vi "Controller - Fire Message.vi"(8 "error in (no error)":errorcluster, 10 "Message Name":T1, 11 "View Model":T2) -> (0 "error out":errorcluster, 3 "View Model":T2)   [LabVIEW 2017]
doc: "Fire message user event with parameters"
uses:
  View Model/Controls/View Model.ctl
  Error Handler/Controls/Error Model.ctl
  Error Handler/Controls/Error Data.ctl
  Error Handler/Controls/Error Type.ctl
  View Model/Controls/Shared Model.ctl
  Configuration/Controls/Config Model.ctl
  Configuration/Controls/Config CMD.ctl
  Configuration/Controls/Config Data.ctl
  Controls/Controller Model.ctl
  Controls/Controller Overhead.ctl
  Controls/Controller States.ctl
  Controls/Controller Message Data.ctl
  Controls/Controller Message Name.ctl
  Views/User Console View/Controls/User Console - Keypad.ctl
  Views/User Console View/Controls/User Console - Transactions.ctl
  Controls/Controller CMD.ctl
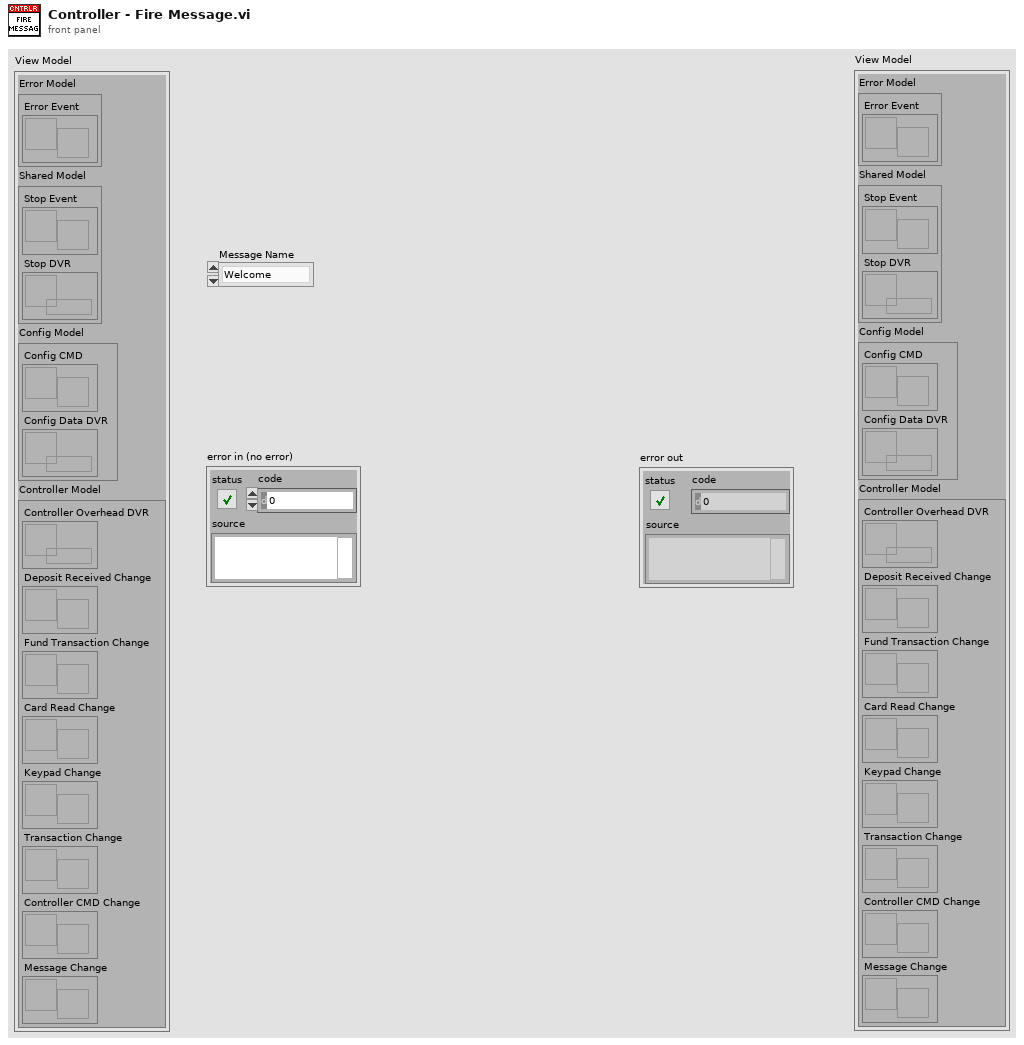
[diagram p1: front panel]
types:
  T1 = typedef "Controller Message Name.ctl" = enum16{"Welcome", "Login", "Idle", "Invalid Login", "Terminate", "Deposit", "Withdrawal", "Fast Cash", "Withdrawal Complete", "Withdrawal Failed", "Balance Inquiry"}
  T2 = typedef "View Model.ctl" = cluster{"Error Model":T3, "Shared Model":T4, "Config Model":T5, "Controller Model":T6}
  T3 = typedef "Error Model.ctl" = cluster{"Error Event":refnum<user-event>}
  T4 = typedef "Shared Model.ctl" = cluster{"Stop Event":refnum<user-event>, "Stop DVR":refnum<data-value>}
  T5 = typedef "Config Model.ctl" = cluster{"Config CMD":refnum<user-event>, "Config Data DVR":refnum<data-value>}
  T6 = typedef "Controller Model.ctl" = cluster{"Controller Overhead DVR":refnum<data-value>, "Deposit Received Change":refnum<user-event>, "Fund Transaction Change":refnum<user-event>, "Card Read Change":refnum<user-event>, "Keypad Change":refnum<user-event>, "Transaction Change":refnum<user-event>, "Controller CMD Change":refnum<user-event>, "Message Change":refnum<user-event>}
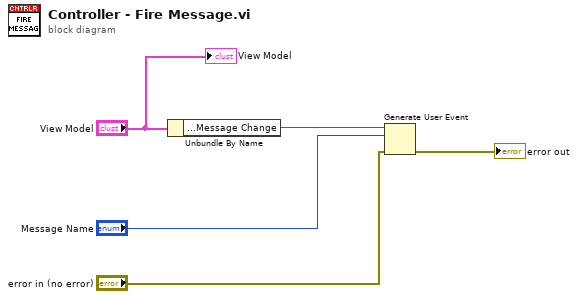
[diagram p0: block diagram]
diagram:
  n1 = Unbundle By Name("View Model") -> ("Controller Model.Message Change"=w5:refnum<user-event>)
  n2 = Generate User Event(user event=w5, event data cluster="Message Name", error in="error in (no error)") -> (error out=→"error out":errorcluster)  [unwired: 1 in, 1 out]
  "View Model" <- "View Model"
